vi "Neocera Simulate Manual Heater.vi"(8 "error in (no error)":errorcluster, 11 "Instrument VISA address":refnum<visa-resource-name>="GPIB0::15::INSTR") -> (0 "error out":errorcluster, 3 "Instrument VISA address out":refnum<visa-resource-name>="GPIB0::15::INSTR")   [LabVIEW 2015]
panel:
  out "read buffer":string
  in  "Heater power, %":dbl
  in  "Set point":dbl=300.0
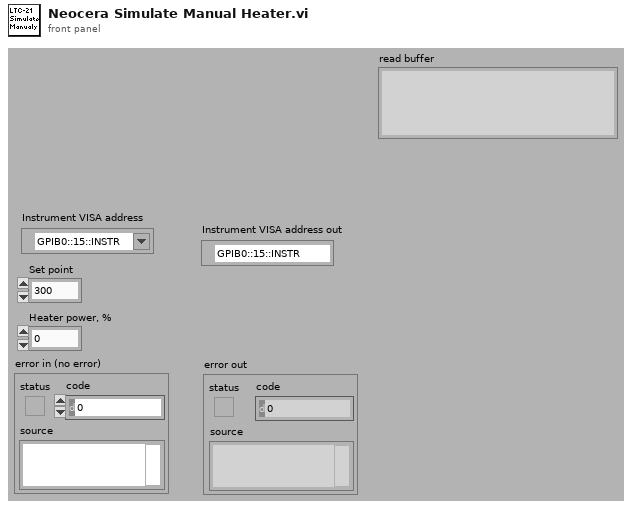
[diagram p1: front panel]
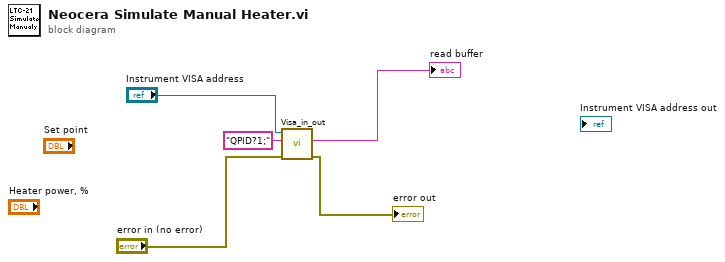
[diagram p0: block diagram]
diagram:
  n1 = call "Visa_in_out.vi"("error in (no error)"="error in (no error)", "write buffer"="QPID?1;", "VISA resource name"="Instrument VISA address") -> ("error out"=→"error out":errorcluster, "read buffer"=→"read buffer":string)  [unwired: 6 in, 1 out]
